vi "string concatition.vi"() -> ()   [LabVIEW 2025]
panel:
  out "subset string":string
  out "reverse string":string
  in  "input String 3":string
  out "concatination":string
  in  "input String 2":string
  out "string length":dbl
  in  "input String":string
  # "offset = on which  is to be started after chars"
  # "length= up to which index to be print the sting of the index"
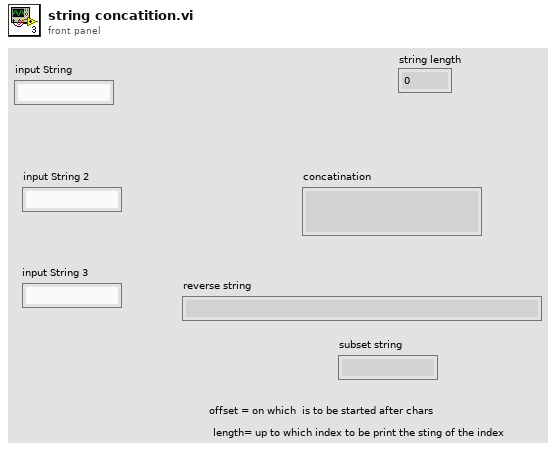
[diagram p1: front panel]
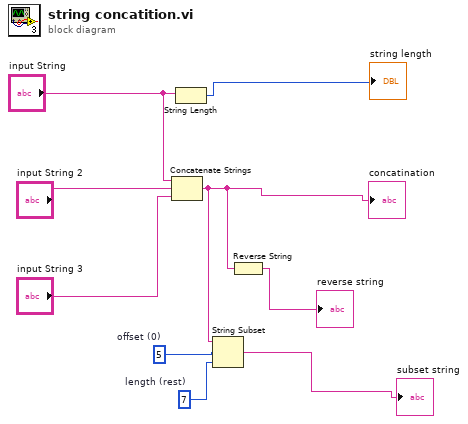
[diagram p0: block diagram]
diagram:
  w2 = 7  # length (rest)
  w3 = 5  # offset (0)
  n1 = Concatenate Strings("input String", "input String 2", "input String 3") -> (w5:string)
  "concatination" <- w5
  n2 = String Length(string="input String") -> (length=→"string length":i32)
  n3 = String Subset(string=w5, offset (0)=w3, length (rest)=w2) -> (substring=→"subset string":string)
  n4 = Reverse String(1:w5) -> (0:→"reverse string":string)
